vi "Configure Waveform.vi"(7 "Waveform Type":T2, 8 "error in (no error)":errorcluster, 9 "Waveform Properties":T1, 10 "Channel(s)":i32[](array[numeric]), 11 "PXIe5413 in":refnum<class "PXIe5413.lvclass">) -> (0 "error out":errorcluster, 3 "PXIe5413 out":refnum<class "PXIe5413.lvclass">)   [LabVIEW 2018, in "PXIe5413.lvlib" / "PXIe5413.lvclass"]
uses:
  PXIe5413.lvclass
  PPLs/Function Generator/Parent/Function Generator.lvlibp/Custom Controls/Waveform Type.ctl
  PPLs/Function Generator/Parent/Function Generator.lvlibp/Custom Controls/Waveform Properties.ctl
  <instrlib>/niFgen/niFgen.llb/niFgen Waveform Type.ctl
  PPLs/Function Generator/Parent/Function Generator.lvlibp/Function Generator.lvclass
  C:/Projects/LabVIEW/PPLs/Function Generator/Parent/Function Generator.lvlibp/Function Generator.lvclass
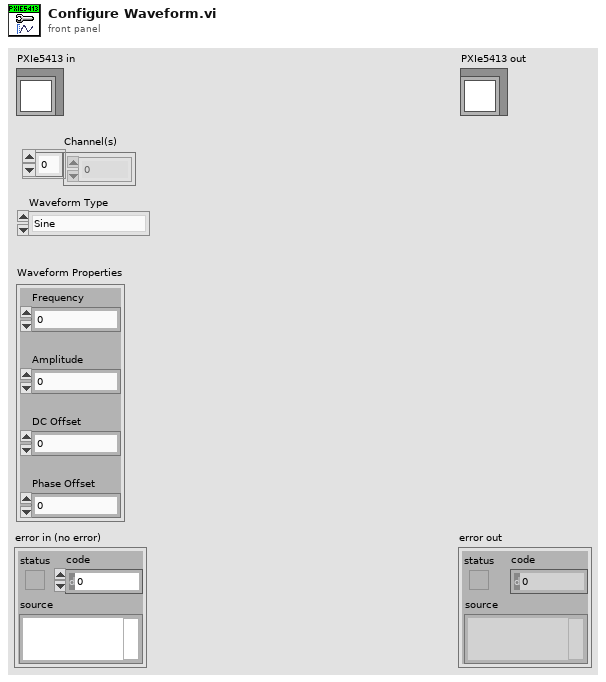
[diagram p1: front panel]
types:
  T1 = typedef "Function Generator.lvlibp/Function Generator.lvclass/Waveform Properties.ctl" = cluster{"Frequency":dbl, "Amplitude":dbl, "DC Offset":dbl, "Phase Offset":dbl}
  T2 = typedef "Function Generator.lvlibp/Function Generator.lvclass/Waveform Type.ctl" = enum16{"Sine", "Square", "Triangle", "Ramp Up", "Ramp Down", "DC", "Noise", "User-Defined"}
  T3 = typedef "niFgen Waveform Type.ctl" = i32
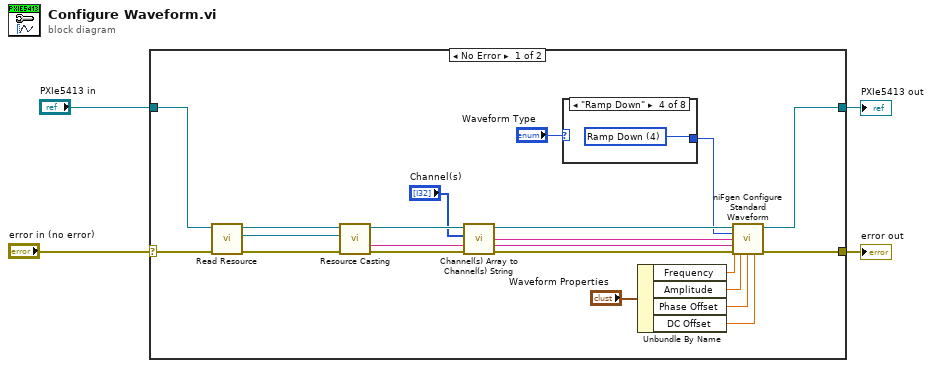
[diagram p0: block diagram]
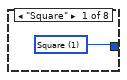
[diagram p2: hidden frame]
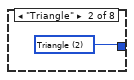
[diagram p3: hidden frame]
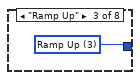
[diagram p4: hidden frame]
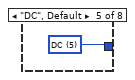
[diagram p5: hidden frame]
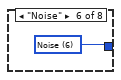
[diagram p6: hidden frame]
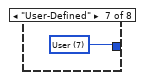
[diagram p7: hidden frame]
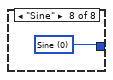
[diagram p8: hidden frame]
diagram:
  n1 = case shown="No Error" "error in (no error)" {
    selector: "error in (no error)" -> [w24 w34]
    tunnel: [w14 w34] -> w3
    tunnel: [w8 w33] -> w2
    tunnel: "PXIe5413 in" -> [w23 w33]
    frame No Error {
      n2 = call "Read Resource.vi"("error in (no error)"=w24, "Function Generator in"=w23) -> ("error out"=w22:errorcluster, "Resource"=w5:refnum<visa-resource-name>, "Function Generator out"=w21:refnum<class "PXIe5413.lvclass">)  [unwired: 7 in]
      n3 = call "Resource Casting.vi"("error in (no error)"=w22, "VISA Resource In"=w5, "PXIe5413 in"=w21) -> ("error out"=w20:errorcluster, "Casted Resource"=w19:string, "PXIe5413 out"=w17:refnum<class "PXIe5413.lvclass">)  [unwired: 6 in]
      n4 = call "Channel(s) Array to Channel(s) String.vi"("error in (no error)"=w20, "Channel(s)"="Channel(s)", "PXIe5413 in"=w17) -> ("error out"=w18:errorcluster, "Channels String"=w15:string, "PXIe5413 out"=w8:refnum<class "PXIe5413.lvclass">)  [unwired: 6 in]
      n5 = case shown="\"Ramp Down\"" "Waveform Type" {
        tunnel: [w25 w26 w27 w28 w29 w30 w31 w32] -> w6
        frame "Square" {
          w25 = T3 1 items=["Sine", "Square", "Triangle", "Ramp Up", "Ramp Down", "DC", "Noise", "User"] ("Waveform")
        }
        frame "Triangle" {
          w26 = T3 2 items=["Sine", "Square", "Triangle", "Ramp Up", "Ramp Down", "DC", "Noise", "User"] ("Waveform")
        }
        frame "Ramp Up" {
          w27 = T3 3 items=["Sine", "Square", "Triangle", "Ramp Up", "Ramp Down", "DC", "Noise", "User"] ("Waveform")
        }
        frame "Ramp Down" {
          w28 = T3 4 items=["Sine", "Square", "Triangle", "Ramp Up", "Ramp Down", "DC", "Noise", "User"] ("Waveform")
        }
        frame "DC", Default {
          w29 = T3 5 items=["Sine", "Square", "Triangle", "Ramp Up", "Ramp Down", "DC", "Noise", "User"] ("Waveform")
        }
        frame "Noise" {
          w30 = T3 6 items=["Sine", "Square", "Triangle", "Ramp Up", "Ramp Down", "DC", "Noise", "User"] ("Waveform")
        }
        frame "User-Defined" {
          w31 = T3 7 items=["Sine", "Square", "Triangle", "Ramp Up", "Ramp Down", "DC", "Noise", "User"] ("Waveform")
        }
        frame "Sine" {
          w32 = T3 0 items=["Sine", "Square", "Triangle", "Ramp Up", "Ramp Down", "DC", "Noise", "User"] ("Waveform")
        }
      }
      n6 = Unbundle By Name("Waveform Properties") -> ("Frequency"=w12:dbl, "Amplitude"=w11:dbl, "Phase Offset"=w10:dbl, "DC Offset"=w9:dbl)
      n7 = call <instrlib>:"niFgen Configure Standard Waveform.vi"("Instrument Handle"=w19, "Channel Name"=w15, "Waveform"=w6, "Frequency"=w12, "Amplitude"=w11, "error in (no error)"=w18, "Start Phase"=w10, "DC Offset"=w9) -> ("error out"=w14:errorcluster)  [unwired: 6 in, 1 out]
    }
    frame Error {
    }
  }
  "error out" <- w3
  "PXIe5413 out" <- w2
